vi "GSE 350 Main.vi"(7 "Use While Loop?":bool, 8 "Error In":errorcluster, 11 "VISA Refnum in":refnum<visa-resource-name>) -> (0 "Error Out":errorcluster, 2 "Weight (lb/kg)":dbl, 3 "Weight Data":string[][](array[string]))   [LabVIEW 2020]
panel:
  out "read buffer":string
  in  "stop":bool
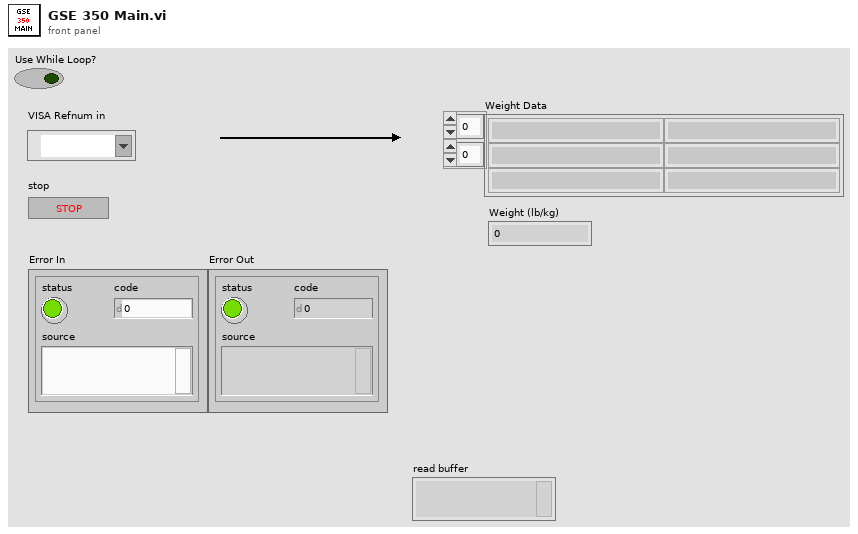
[diagram p1: front panel]
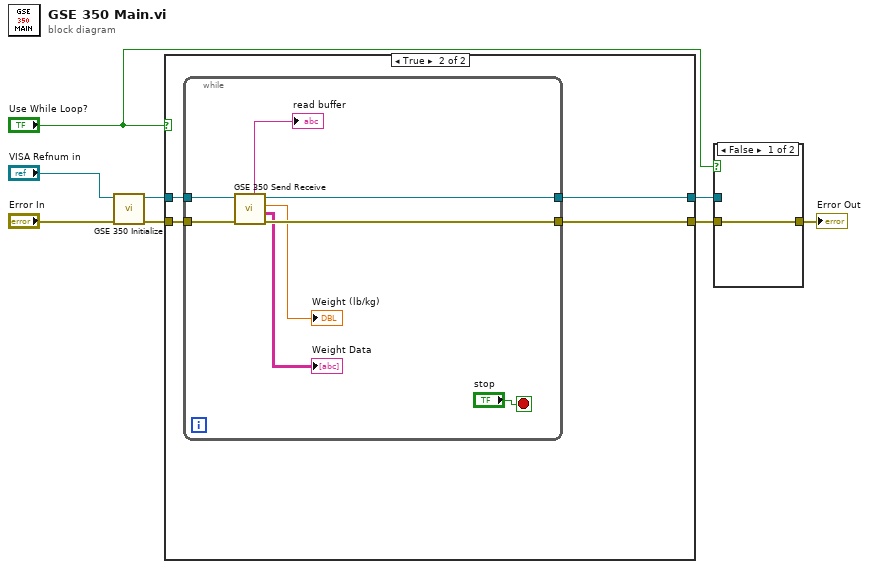
[diagram p0: block diagram]
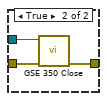
[diagram p2: hidden frame]
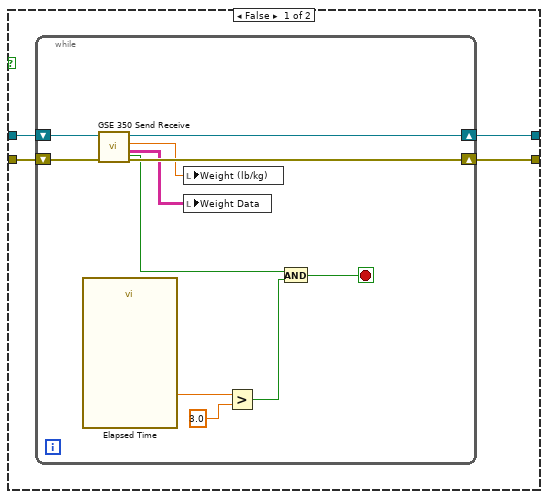
[diagram p3: hidden frame]
diagram:
  n1 = call "GSE 350 Initialize.vi"("error in (no error)"="Error In", "VISA Refnum in"="VISA Refnum in") -> ("error out"=w4:errorcluster, "VISA Refnum out"=w5:refnum<visa-resource-name>)  [unwired: 8 in]
  n2 = case shown="True" "Use While Loop?" {
    tunnel: [w11 w27] -> w8
    tunnel: [w10 w26] -> w7
    tunnel: w5 -> [w12 w25]
    tunnel: w4 -> [w9 w24]
    frame False {
      n3 = while {
        shift-right: [w22] -> w11
        shift-left: w12 -> [w23]
        shift-right: [w21] -> w10
        shift-left: w9 -> [w20]
        stop <- w15 stop-if-true
        n4 = call "Elapsed Time"() -> ("Elapsed Time (s)"=w14:dbl)  [unwired: 12 in, 7 out]
        n5 = call "GSE 350 Send Receive.vi"("error in (no error)"=w20, "VISA Refnum in"=w23) -> ("error out"=w21:errorcluster, "Weight Data"=w18:string[][], "Weight (lb/kg)"=w19:dbl, "VISA Refnum out"=w22:refnum<visa-resource-name>, "Match Found!"=w16:bool)  [unwired: 4 in, 1 out]
        n6 = local write "Weight (lb/kg)"(w19) -> ()
        n7 = local write "Weight Data"(w18) -> ()
        n8 = Greater?(x=w14, y=3.0) -> (0:w17:bool)
        n9 = And(x=w16, y=w17) -> (x .and. y?=w15:bool)
      }
    }
    frame True {
      n10 = while {
        tunnel: [w34] -> w27
        tunnel: [w33] -> w26
        tunnel: w25 -> [w32]
        tunnel: w24 -> [w31]
        stop <- "stop" stop-if-true
        n11 = call "GSE 350 Send Receive.vi"("error in (no error)"=w31, "VISA Refnum in"=w32) -> ("error out"=w33:errorcluster, "Weight Data"=→"Weight Data":string[][], "Weight (lb/kg)"=→"Weight (lb/kg)":dbl, "VISA Refnum out"=w34:refnum<visa-resource-name>, "read buffer"=→"read buffer":string)  [unwired: 4 in, 1 out]
      }
    }
  }
  n12 = case shown="False" "Use While Loop?" {
    tunnel: w8 -> [_ w39]
    tunnel: w7 -> [w36 w38]
    tunnel: [w36 w37] -> w2
    frame False {
    }
    frame True {
      n13 = call "GSE 350 Close.vi"("error in (no error)"=w38, "VISA Refnum in"=w39) -> ("error out"=w37:errorcluster)  [unwired: 9 in]
    }
  }
  "Error Out" <- w2
